vi "XYStage_Move.vi"(0 "Y_Wait":bool=TRUE, 1 "Position Y":sgl, 2 "Position X":sgl, 3 "X_Wait":bool=TRUE) -> ()   [LabVIEW 2016]
uses:
  Utility/Global_Stage.vi
  Utility/Global Constants.vi
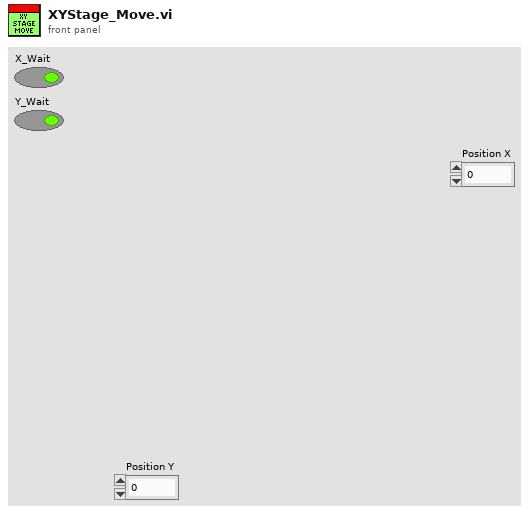
[diagram p1: front panel]
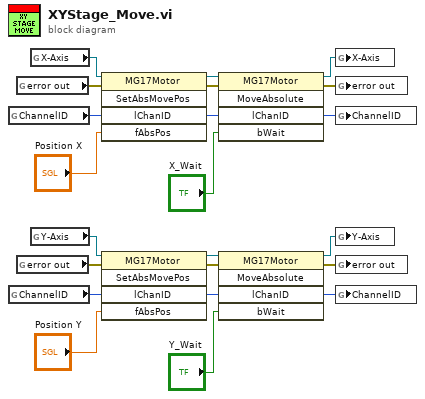
[diagram p0: block diagram]
diagram:
  n1 = global read "Global_Stage.vi" "ChannelID"() -> (w15:i32)
  n2 = global read "Global_Stage.vi" "ChannelID"() -> (w4:i32)
  n3 = global read "Global Constants.vi" "error out"() -> (w14:errorcluster)
  n4 = global read "Global Constants.vi" "error out"() -> (w3:errorcluster)
  n5 = global read "Global_Stage.vi" "X-Axis"() -> (w17:refnum<k7>)
  n6 = global read "Global_Stage.vi" "Y-Axis"() -> (w6:refnum<k7>)
  n7 = invoke class="MG17Motor" method="SetAbsMovePos"(reference=w17, error in=w14, "lChanID"=w15, "fAbsPos"="Position X") -> (reference out=w20:refnum<k7>, error out=w21:errorcluster, "lChanID"=w22:i32)  [unwired: 1 in, 2 out]
  n8 = invoke class="MG17Motor" method="SetAbsMovePos"(reference=w6, error in=w3, "lChanID"=w4, "fAbsPos"="Position Y") -> (reference out=w9:refnum<k7>, error out=w10:errorcluster, "lChanID"=w11:i32)  [unwired: 1 in, 2 out]
  n9 = invoke class="MG17Motor" method="MoveAbsolute"(reference=w20, error in=w21, "lChanID"=w22, "bWait"="X_Wait") -> (reference out=w16:refnum<k7>, error out=w13:errorcluster, "lChanID"=w12:i32)  [unwired: 1 in, 2 out]
  n10 = invoke class="MG17Motor" method="MoveAbsolute"(reference=w9, error in=w10, "lChanID"=w11, "bWait"="Y_Wait") -> (reference out=w5:refnum<k7>, error out=w2:errorcluster, "lChanID"=w1:i32)  [unwired: 1 in, 2 out]
  n11 = global write "Global_Stage.vi" "X-Axis"(w16) -> ()
  n12 = global write "Global Constants.vi" "error out"(w13) -> ()
  n13 = global write "Global_Stage.vi" "ChannelID"(w12) -> ()
  n14 = global write "Global_Stage.vi" "Y-Axis"(w5) -> ()
  n15 = global write "Global Constants.vi" "error out"(w2) -> ()
  n16 = global write "Global_Stage.vi" "ChannelID"(w1) -> ()
